vi "GetSnapshot.vi"(0 "error in":errorcluster) -> (1 "error out":errorcluster, 2 "Status":bool)   [LabVIEW 2014]
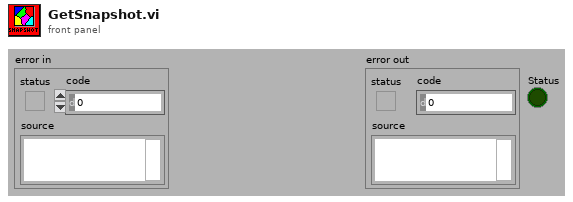
[diagram p1: front panel]
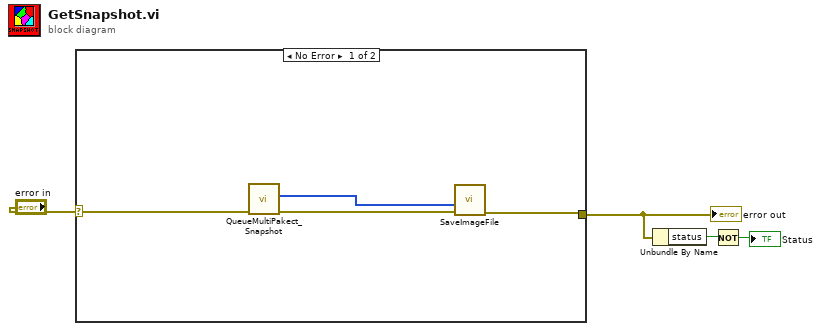
[diagram p0: block diagram]
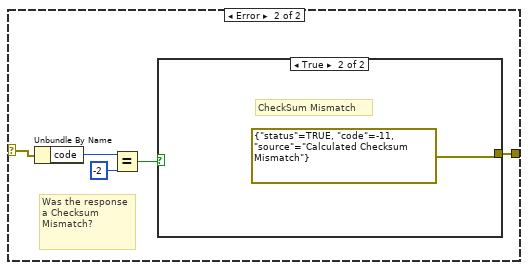
[diagram p2: hidden frame]
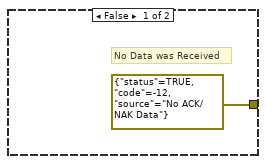
[diagram p3: hidden frame]
diagram:
  n1 = case shown="No Error" "error in" {
    selector: "error in" -> [w8 w12]
    tunnel: [w6 w13] -> w4
    frame No Error {
      n2 = call "QueueMultiPakect_Snapshot.vi"("no error"=w8) -> ("error out"=w7:errorcluster, "ImageData"=w5:u8[])  [unwired: 6 in, 3 out]
      n3 = call "SaveImageFile.vi"("error in"=w7, "ImagData"=w5) -> ("error out"=w6:errorcluster)  [unwired: 7 in, 2 out]
    }
    frame Error {
      # "Was the response a Checksum\nMismatch?"
      n4 = Unbundle By Name(w12) -> ("code"=w11:i32)
      n5 = Equal?(x=w11, y=-2) -> (x = y?=w9:bool)
      n6 = case shown="True" w9 {
        tunnel: [errorcluster {"status"=TRUE, "code"=-12, "source"="No ACK/NAK Data"} ("error out") errorcluster {"status"=TRUE, "code"=-11, "source"="Calculated Checksum Mismatch"} ("error out")] -> w13
        frame False {
          # "No Data was Received"
        }
        frame True {
          # "CheckSum Mismatch"
        }
      }
    }
  }
  "error out" <- w4
  n7 = Unbundle By Name(w4) -> ("status"=w3:bool)
  n8 = Not(x=w3) -> (.not. x?=→"Status":bool)
